vi "DataStream_RT_Create.vi"() -> (0 "Error Out":errorcluster, 3 "Stream Writer Ref Out":T1)   [LabVIEW 2020]
uses:
  TypeDefs/Cluster_DataStream_RT Writer Refs.ctl
  <vilib>/dex/Stream Element Allocation Mode.ctl
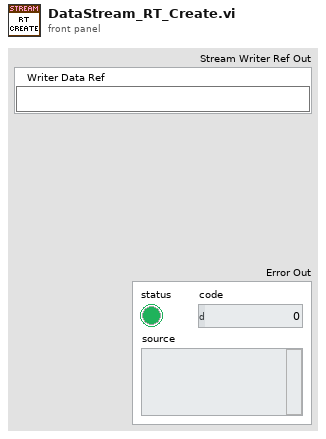
[diagram p1: front panel]
types:
  T1 = typedef "Cluster_DataStream_RT Writer Refs.ctl" = cluster{"Writer Data Ref":refnum<k21>}
  T2 = typedef "Stream Element Allocation Mode.ctl" = u32
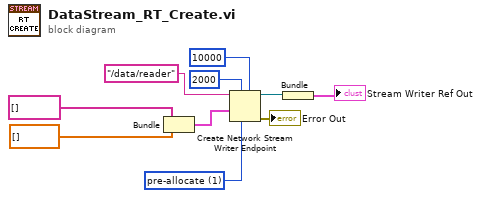
[diagram p0: block diagram]
diagram:
  w10 = T2 1 items=["allocate as needed", "pre-allocate"] ("element allocation mode")
  n1 = Bundle(string[] [], dbl[] []) -> (w3:cluster{string[], dbl[]})  [unwired: 1 in]
  n2 = Create Network Stream Writer Endpoint(5:10000 ("timeout in ms (-1)"), 6:w10, 7:2000 ("reader buffer size"), 9:w3, 11:"/data/reader" ("writer name")) -> (0:→"Error Out":errorcluster, 3:w6:refnum<k21>)  [unwired: 2 in]
  n3 = Bundle("writer name"=w6) -> (→"Stream Writer Ref Out":cluster{"writer name":refnum<k21>})  [unwired: 1 in]
